vi "Get SubpanelVI Info.vi"(8 "error in (no error)":errorcluster, 11 "DispSnsr Configuration in":refnum<class "DispSnsr Configuration.lvclass">) -> (0 "error out":errorcluster, 1 "Subpanel VI data":T1, 2 "Category string":string, 3 "DispSnsr Configuration out":refnum<class "DispSnsr Configuration.lvclass">)   [LabVIEW 2016, in "Hardware.lvlib" / "Displacement Sensor.lvlib" / "DispSnsr Configuration.lvclass"]
uses:
  <userlib>/Common Components/Hardware/Displacement Sensor/DispSnsr Config/DispSnsr Configuration.lvclass
  <userlib>/Configuration Dialog Actor/Methods/Data Retrieved by Lookup Table.ctl
  <userlib>/Configuration Dialog Actor/Configuration.lvclass
  <userlib>/Common Components/Hardware/Displacement Sensor/DispSnsr Config/DispSnsr Configuration.lvclass/DispSnsr Configuration.ctl
  <userlib>/Common Components/Hardware/Abstract Hardware/Hardware.lvclass/Hardware.ctl
  <userlib>/Common Components/Hardware/Abstract Hardware/Read Label.vi
  <userlib>/Common Components/Hardware/Displacement Sensor/DispSnsr/DispSnsr.lvclass
  C:/Program Files (x86)/National Instruments/LabVIEW 2016/user.lib/Common Components/Hardware/Abstract Hardware/Hardware.lvclass
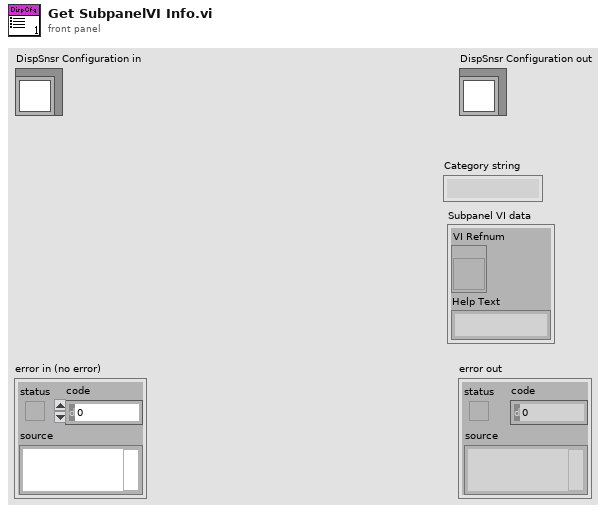
[diagram p1: front panel]
types:
  T1 = typedef "Configuration.lvlib/Configuration.lvclass/Data Retrieved by Lookup Table.ctl" = cluster{"VI Refnum":refnum<vi>, "Help Text":string}
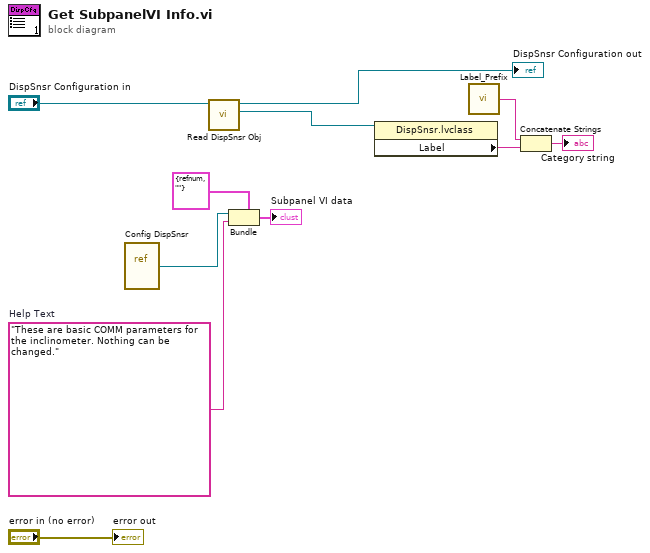
[diagram p0: block diagram]
diagram:
  w3 = "These are basic COMM parameters for the inclinometer. Nothing can be changed."  # Help Text
  n1 = vi-ref <userlib>:"Config DispSnsr.vi"() -> (w4:refnum<vi>)
  n2 = call <userlib>:"Read DispSnsr Obj.vi"("DispSnsr Configuration in"="DispSnsr Configuration in") -> ("Hardware.lvlib:Displacement Sensor.lvlib:DispSnsr.lvclass"=w9:refnum<class "DispSnsr.lvclass">, "DispSnsr Configuration out"=→"DispSnsr Configuration out":refnum<class "DispSnsr Configuration.lvclass">)  [unwired: 9 in]
  n3 = Bundle(cluster=T1 {"VI Refnum"=refnum, "Help Text"=""} ("output cluster"), "VI Refnum"=w4, "Help Text"=w3) -> (→"Subpanel VI data":T1)
  n4 = property class="DispSnsr.lvclass"(reference=w9) -> ("Label"=w1:string)  [unwired: 1 in, 2 out]
  n5 = call <userlib>:"Label_Prefix.vi"() -> ("Label Prefix String"=w10:string)
  n6 = Concatenate Strings(w10, w1) -> (→"Category string":string)
  "error out" <- "error in (no error)"
